vi "Find Device.vi"   [LabVIEW 2013, in "ACNET Monitor.lvlib"]
uses:
  ACNET Monitor.lvlib
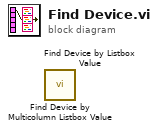
[diagram p0: block diagram]
diagram:
  n1 = call "Find Device by Multicolumn Listbox Value.vi"() -> ()  [unwired: 3 in, 3 out]
  n2 = call "Find Device by Listbox Value.vi"() -> ()  [unwired: 3 in, 3 out]
